vi "Setup Select Unwired Button.vi"(7 "Action":T2, 9 "Display Items":T1[](array[typedef]), 10 "Properties for Tree In":T3(array[cluster]), 11 "Boolean in":refnum<vi>) -> ()   [LabVIEW 2023]
uses:
  controls/action enum.ctl
  cluster/Cluster Element Description.ctl
panel:
  # "OR"
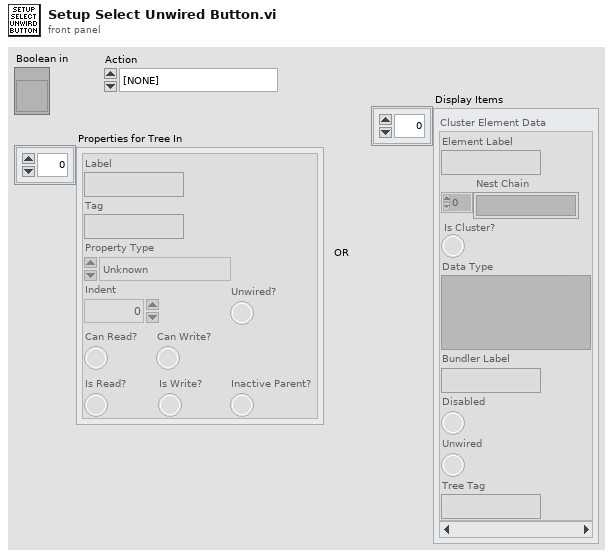
[diagram p1: front panel]
types:
  T1 = typedef "Cluster Element Description.ctl" = cluster{"Element Label":string, "Nest Chain":string[], "Is Cluster?":bool, "Data Type":variant, "Bundler Label":string, "Disabled":bool, "Unwired":bool, "Tree Tag":string}
  T2 = typedef "action enum.ctl" = enum16{"[NONE]", "Wire Bundle", "Wire Unbundle", "Terminal Unbundle", "Terminal Bundle", "Bundler Move Up", "Bundler Move Down", "Bundler Insert", "Bundler Remove", "Bundler Remove Unwired", "Bundler Rearrange", "In Place Insert", "In Place Remove", "In Place Remove Unwired", "In Place Rearrange", "Wire Properties", "Wire Method", "Terminal Properties", "Terminal Method", "Property Move Up", "Property Move Down", "Properties Insert", "Properties Remove", "Properties Remove Unwired", "Properties Rearrange", "Method Change", "Class for Constant", "Class For Control", "Class For Node", "Class Name to Clipboard"}
  T3 = cluster{"Label":string, "Tag":string, "Property Type":enum16{"Unknown", "Base", "Scripting", "Private", "Deprecated", "None", "Divider"}, "Indent":u16, "Can Read?":bool, "Can Write?":bool, "Is Read?":bool, "Is Write?":bool, "Inactive Parent?":bool, "Unwired?":bool}[]
  T4 = enum8{"Enabled", "Disabled", "Disabled and Grayed Out"}
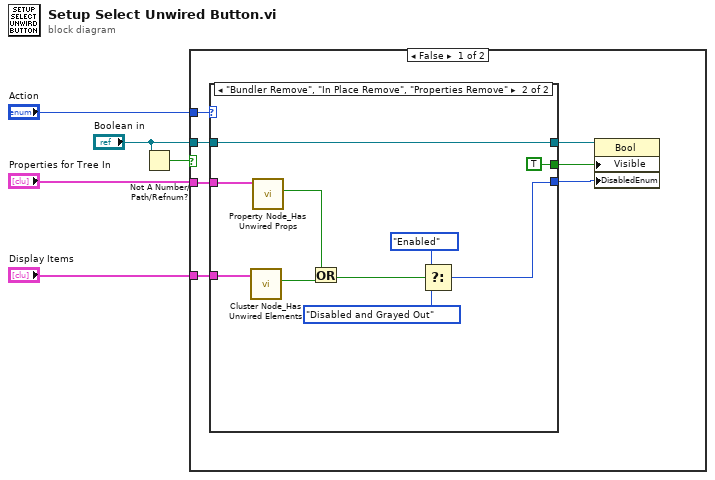
[diagram p0: block diagram]
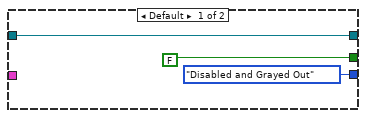
[diagram p2: hidden frame]
diagram:
  n1 = Not A Number/Path/Refnum?(number/path/refnum="Boolean in") -> (NaN/Path/Refnum?=w5:bool)
  n2 = case shown="False" w5 {
    tunnel: "Boolean in" -> [w11 _]
    tunnel: "Action" -> [w10 _]
    tunnel: "Properties for Tree In" -> [w8 _]
    tunnel: "Display Items" -> [w7 _]
    frame False {
      n3 = case shown="\"Bundler Remove\", \"In Place Remove\", \"Properties Remove\"" w10 {
        tunnel: [w14 w25] -> w12
        tunnel: w11 -> [w14 w25]
        tunnel: [FALSE TRUE] -> w9
        tunnel: w8 -> [_ w24]
        tunnel: w7 -> [_ w23]
        tunnel: [T4."Disabled and Grayed Out" ("Disabled") w17] -> w6
        frame Default {
        }
        frame "Bundler Remove", "In Place Remove", "Properties Remove" {
          n4 = call "Cluster Node_Has Unwired Elements.vi"("Display Items"=w23) -> ("Has unwired properties?"=w22:bool)  [unwired: 9 in, 1 out]
          n5 = call "Property Node_Has Unwired Props.vi"("Properties for Tree In"=w24) -> ("Has unwired properties?"=w21:bool)  [unwired: 9 in, 1 out]
          n6 = Or(x=w21, y=w22) -> (x .or. y?=w18:bool)
          n7 = Select(t=T4."Enabled" ("Disabled"), s=w18, f=T4."Disabled and Grayed Out" ("Disabled")) -> (s? t:f=w17:T4)
        }
      }
      n8 = property class="Bool"(reference=w12, "Visible"=w9, "DisabledEnum"=w6) -> ()  [unwired: 1 in, 2 out]
    }
    frame True {
    }
  }
